vi "XYZStage-Monitor move execution.vi"(8 "error in (no error)":errorcluster, 10 "XYZ Position Command Output":T1 {"XYZ Coordinates"."Z" format="Z= %#_g"; "XYZ Coordinates"."Y" format="Y= %#_g"; "XYZ Coordinates"."X" format="X= %#_g"; "Z Limit (um+/-)" format="Z Limit = %.0f"; "Speed" format="Speed= %.0f"}, 11 "XYZ Stage Control in":refnum<class "XYZ Stage Control.lvclass">) -> (0 "error out":errorcluster, 1 "Time has Elapsed":bool, 2 "Motor E-stop":bool, 3 "XYZ Stage Control out":refnum<class "XYZ Stage Control.lvclass">, 4 "Position reached":bool)   [LabVIEW 2020]
uses:
  XYZ Stage Control/XYZ Stage Control.lvclass
  XYZ Stage Control/typedefs/XYZ_position_input.ctl
  XYZ Stage Control/typedefs/XYZ axes.ctl
  Typedefs/XYZ_coordinates.ctl
  Global Variables/gl_UI Ctrl Refs.vi
  User Interface/Windows/Position control window/Globals/Pos ctrl window globals.vi
  Globals/gl_XYZStage globals.vi
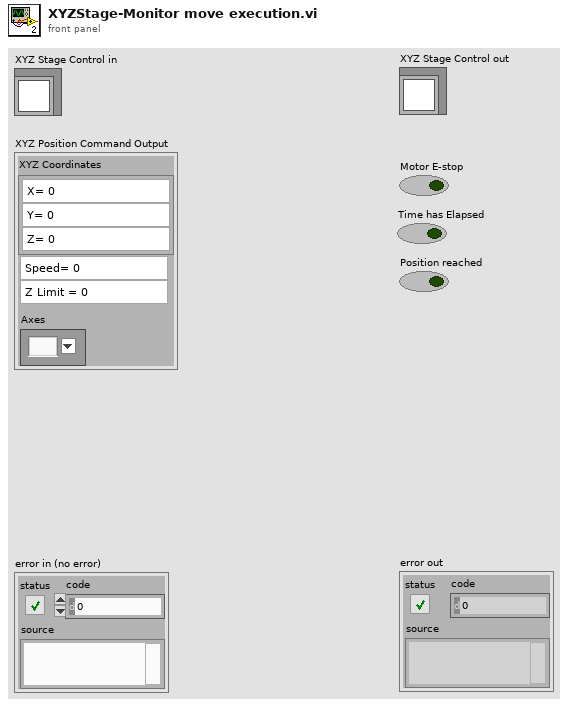
[diagram p1: front panel]
types:
  T1 = typedef "XYZ_position_input.ctl" = cluster{"Speed":i32, "Z Limit (um+/-)":sgl, "Axes":T2, "XYZ Coordinates":T3}
  T2 = typedef "XYZ axes.ctl" = string
  T3 = typedef "XYZ_coordinates.ctl" = cluster{"X":sgl, "Y":sgl, "Z":sgl}
  T4 = typedef "UI ctrl refs cluster.ctl" = cluster{"Top level VI path":path, "Top level VI ref":refnum<vi>, "User menu ref":refnum<k9>, "Sub Panel control":refnum<vi>, "Imaging Param Tab":refnum<vi>, "Occurrence-Start drivers":refnum<k4>, "Occurrence-Speed logging initialised":refnum<k4>, "Occurrence-XYZ stage initialised":refnum<k4>, "Exit button":refnum<vi>, "Status ind":refnum<vi>, "Set as origin":refnum<vi>, "Speed Logging":refnum<vi>, "Time Lapse":refnum<vi>, "Live Imaging":refnum<vi>, "AOL Z Stack":refnum<vi>, "Motor Z Stack":refnum<vi>, "Funct Acq button":refnum<vi>, "Hard Shutter":refnum<vi>, "Virtual Shutter":refnum<vi>, "Laser Power":refnum<vi>, "AOL Mode":refnum<vi>, "Frame Size":refnum<vi>, "Field of View":refnum<vi>, "Dwell Time":refnum<vi>, "Zoom":refnum<vi>, "AOL Z":refnum<vi>, "Objective":refnum<vi>, "Axis":refnum<vi>, "Paths & Names":refnum<vi>, "Experiment folder path (ind.)":refnum<vi>, "Last State (Ind.)":refnum<vi>, "Averages":refnum<vi>, "Angle (degrees)":refnum<vi>, "X centre":refnum<vi>, "Y centre":refnum<vi>, "Plane Mode":refnum<vi>, "# Planes":refnum<vi>, "Z Start":refnum<vi>, "Z Stop":refnum<vi>, "Z Step":refnum<vi>, "PMT 1":refnum<vi>, "PMT 2":refnum<vi>, "Stage XYZ Position":refnum<vi>, "Pockels@Z Start":refnum<vi>, "Pockels@Z Stop":refnum<vi>, "Obtain Z Start":refnum<vi>, "Obtain Z Stop":refnum<vi>, "Live stim.trig.period":refnum<vi>, "Live stim.trig.enable":refnum<vi>, "Movement Correction":refnum<vi>, "Load Reference Image":refnum<vi>, "XY Stage Move":refnum<vi>, "MovCor Cluster":refnum<vi>, "RefDAQParam":refnum<vi>, "Funct. Acq. Pockels Modulation":refnum<vi>, "Ref Laser Power":refnum<vi>, "Enable Video Recording":refnum<vi>, "Video Record-Live Imaging":refnum<vi>, "Video Record-Funct acq":refnum<vi>, "Reference Source":refnum<vi>, "AOL Z-stack Chirps Ready (ind)":refnum<vi>, "Target time between mov.cor. ref triggers (ms)":refnum<vi>, "Funct. Acq. Ref frame save":refnum<vi>, "Tracking button":refnum<vi>, "Show ref plots window":refnum<vi>, "Center freq ind (nm)":refnum<vi>, "Pickup mode (ind)":refnum<vi>, "Logging queue (ind)":refnum<vi>, "Back aperture power (ind.)":refnum<vi>, "Power after objective (ind.)":refnum<vi>, "Switch user":refnum<vi>, "Ls1 Conn. Status":refnum<vi>, "Ls1Tuning Status":refnum<vi>, "Ls1 Faults":refnum<vi>, "Ls1 Connection":refnum<vi>, "Ls1 Mode":refnum<vi>, "Ls1 POWER [mW]":refnum<vi>, "Ls1Shutter":refnum<vi>, "Ls1 Wavelength":refnum<vi>, "Ls1 Note":refnum<vi>, "Ls1 Confirm Wav":refnum<vi>, "Ls1 PreChrp Prism1":refnum<vi>, "Ls1 PreChrp Prism2":refnum<vi>, "Ls1 wav top Ind":refnum<vi>, "Ls1 power top Ind":refnum<vi>, "Ls1 Pump peak Hold":refnum<vi>, "Ls1 Status Ind":refnum<vi>, "Ls1 wav cancel":refnum<vi>, "Experiment Type":refnum<vi>, "Biology Information":refnum<vi>, "Camera recording status":refnum<vi>, "Optimise Obj. Pos.":refnum<vi>}
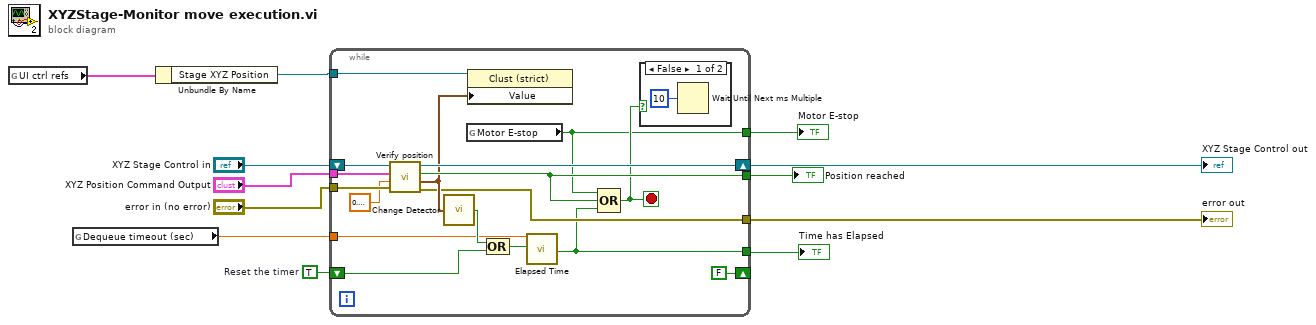
[diagram p0: block diagram]
diagram:
  w8 = TRUE  # Reset the timer
  n1 = global read "gl_UI Ctrl Refs.vi" "UI ctrl refs"() -> (w3:T4)
  n2 = global read "Pos ctrl window globals.vi" "Dequeue timeout (sec)"() -> (w1:dbl)
  n3 = Unbundle By Name(w3) -> ("Stage XYZ Position"=w2:refnum<vi>)
  n4 = while {
    tunnel: "error in (no error)" -> [w28]
    tunnel: "XYZ Position Command Output" -> [w27]
    shift-right: [w25] -> w6
    shift-left: "XYZ Stage Control in" -> [w29]
    tunnel: [w23] -> w7
    tunnel: w2 -> [w24]
    tunnel: w1 -> [w17]
    shift-right: [FALSE ("Reset the timer")] -> _
    shift-left: w8 -> [w16]
    tunnel: [w13] -> w11
    tunnel: [w15] -> w10
    tunnel: [w14] -> w12
    stop <- w21 stop-if-true
    n5 = call-dynamic "Verify position.vi"("error in (no error)"=w28, "Tolerance (um)"=sgl 0.4, "XYZ Position Input"=w27, "XYZ Stage Control in"=w29) -> ("error out"=w14:errorcluster, "XYZ Coordinates"=w22:T3, "Position reached"=w23:bool, "XYZ Stage Control out"=w25:refnum<class "XYZ Stage Control.lvclass">)  [unwired: 4 in]
    n6 = call <userlib>:"Change Detector.vi"("Value"=w22) -> ("Changed?"=w18:bool)
    n7 = global read "gl_XYZStage globals.vi" "Motor E-stop"() -> (w15:bool)
    n8 = property on="Property Node" class="Clust (strict)"(reference=w24, "Value"=w22) -> ()  [unwired: 1 in, 2 out]
    n9 = Compound Arithmetic op=OR(w18, w16) -> (w19:bool)
    n10 = call "Elapsed Time"("Time Target (s)"=w17, "Reset"=w19) -> ("Time has Elapsed"=w13:bool)  [unwired: 10 in, 7 out]
    n11 = Compound Arithmetic op=OR(w15, w23, w13) -> (w21:bool)
    n12 = case shown="False" w21 {
      frame False {
        n13 = Wait Until Next ms Multiple(millisecond multiple=u32 10) -> ()  [unwired: 1 out]
      }
      frame True {
        # "No wait if position reached"
      }
    }
  }
  "error out" <- w12
  "Time has Elapsed" <- w11
  "Motor E-stop" <- w10
  "Position reached" <- w7
  "XYZ Stage Control out" <- w6
